vi "Add Header To LogFile.vi"(8 "Error In":errorcluster, 10 "Header":string[](array[string]), 11 "LogClass In":refnum<class "Logs.lvclass">) -> (0 "Error Out":errorcluster, 3 "LogClass Out":refnum<class "Logs.lvclass">)   [LabVIEW 2019, in "Logs.lvclass"]
uses:
  Logs.lvclass
  3d254321-69f1-4726-a578-02ff3ee58a15.vi
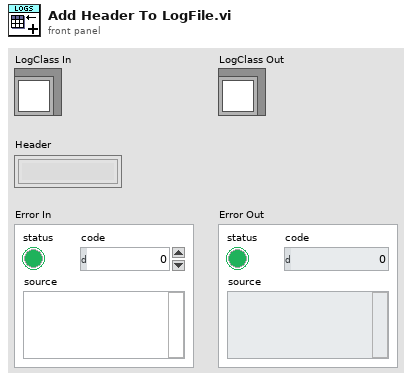
[diagram p1: front panel]
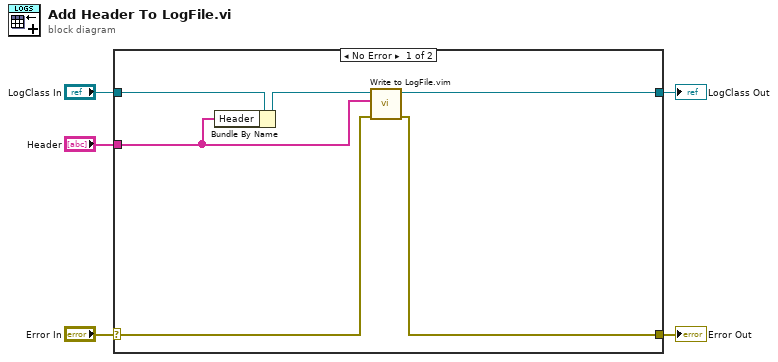
[diagram p0: block diagram]
diagram:
  n1 = case shown="No Error" "Error In" {
    selector: "Error In" -> [w9 w12]
    tunnel: [w8 w12] -> w4
    tunnel: "LogClass In" -> [w11 w13]
    tunnel: "Header" -> [w6 _]
    tunnel: [w10 w13] -> w1
    frame No Error {
      n2 = Bundle By Name(cluster=w11, "Header"=w6) -> (w7:refnum<class "Logs.lvclass">)
      n3 = call "Write to LogFile.vim"("Error In"=w9, "Data"=w6, "LogClass In"=w7) -> ("Error out"=w8:errorcluster, "LogClass Out"=w10:refnum<class "Logs.lvclass">)  [unwired: 7 in]
    }
    frame Error {
    }
  }
  "LogClass Out" <- w1
  "Error Out" <- w4
